vi "Update UI.vi"(8 "error in (no error)":errorcluster, 10 "DataExchange":T1, 11 "Controller Template in":refnum<class "DemoCameraController.lvclass">) -> (0 "error out":errorcluster, 3 "Controller Template out":refnum<class "DemoCameraController.lvclass">)   [LabVIEW 2020, in "DemoCameraController.lvlib" / "DemoCameraController.lvclass"]
uses:
  DemoCameraController.lvclass
  Model/Hardware Abstraction Layer/Component/Device/Device/DataExchange.ctl
  <vilib>/vision/Image Controls.llb/IMAQ Image.ctl
  DemoCameraController.lvclass/DemoCameraController.ctl
  Interface/DataListener/DataListener.lvclass
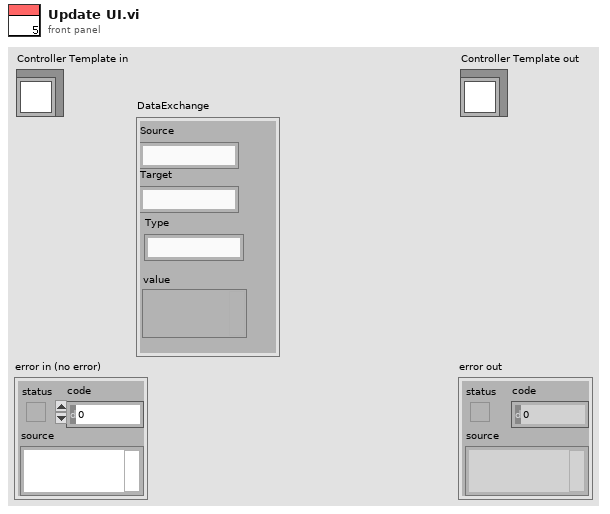
[diagram p1: front panel]
types:
  T1 = typedef "DataListener.lvclass/DataExchange.ctl" = cluster{"Source":string, "Target":string, "Type":string, "value":variant}
  T2 = typedef "IMAQ Image.ctl" = refnum<image>
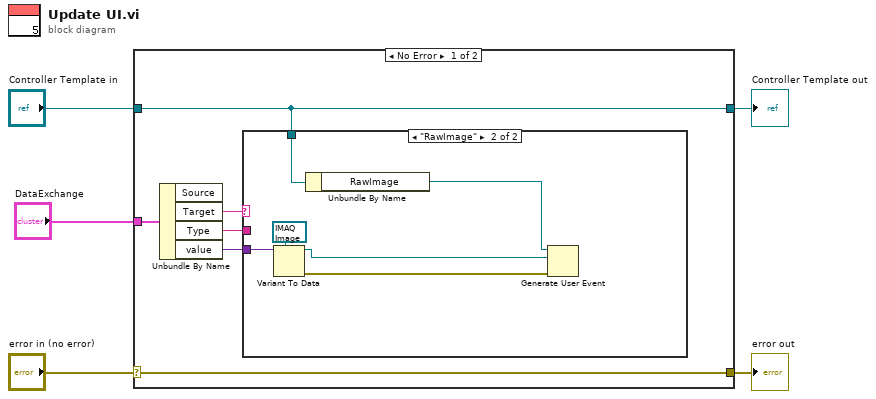
[diagram p0: block diagram]
diagram:
  n1 = case shown="No Error" "error in (no error)" {
    selector: "error in (no error)" -> [w11 w19]
    tunnel: [w11 w19] -> w4
    tunnel: [w6 w18] -> w2
    tunnel: "Controller Template in" -> [w6 w18]
    tunnel: "DataExchange" -> [w10 _]
    frame No Error {
      n2 = Unbundle By Name(w10) -> ("Target"=w7:string, "Type"=w8:string, "value"=w9:variant)  [unwired: 1 out]
      n3 = case shown="\"RawImage\"" w7 {
        tunnel: w9 -> [_ w17]
        tunnel: w8 -> [_ _]
        tunnel: w6 -> [_ w16]
        frame "False", Default {
        }
        frame "RawImage" {
          n4 = Variant To Data(type=T2 refnum ("event data"), Variant=w17) -> (data=w12:T2, error out=w14:errorcluster)  [unwired: 1 in]
          n5 = Unbundle By Name(w16) -> ("RawImage"=w15:refnum<user-event>)
          n6 = Generate User Event(user event=w15, event data cluster=w12, error in=w14) -> ()  [unwired: 1 in, 2 out]
        }
      }
    }
    frame Error {
    }
  }
  "error out" <- w4
  "Controller Template out" <- w2
